vi "Adaptive Channel Equalization.vi"() -> ()   [LabVIEW 2019]
doc: "This example demonstrates how to apply an RLS adaptive filter to channel equalization applications. This example simulates a communication channel with an FIR filter and additional Gaussian noise, simulates the received symbols by applying the FIR filter to the transmitted symbols, and uses an RLS adaptive filter to compensate for the distortion caused by the communication channel. \n\nComplete the following steps to use this example.\n\n1. Select <b>Training</b> from the <b>Mode</b> pull-down menu.\n\n2. Run this example.\n\n3. Observe the <b>Equalizer Output</b> graph until the symbols converge to the four transmitted symbols indicated in the <b>Transmitted Symbols</b> graph.\n\n4. Compare the <b>Equalizer Output</b> and the <b>Received Symbols</b> plot. Notice that the equalizer output converges to the transmitted symbols, whereas the received symbols are difficult to recognize.\n\n5. Select <b>Dicision-Directed</b> from the <b>Mode</b> pull-down menu.\n\n6. Observe the <b>Equalizer Output</b> plot. The equalizer output shows a better convergence."
uses:
  <vilib>/addons/Adaptive Filters/Create/AFT Create FIR RLS (Complex).vi
  <vilib>/addons/Adaptive Filters/Processing/AFT Filter Signal and Update Coefficients (Complex, PtByPt).vi
  <vilib>/addons/Adaptive Filters/Processing/AFT Filter Signal (Complex, PtByPt).vi
  <vilib>/addons/Adaptive Filters/Processing/AFT Update Coefficients (Complex, PtByPt).vi
  <vilib>/addons/Adaptive Filters/NI_AdaptiveFilter.lvlib
panel:
  in  "Tab Control":enum32{"Background", "Scatter Diagram"}(tab)
  in  "Mode":enum16{"Training", "Decision-Directed"}(ring)
  out "Transmitted Symbols":cluster{dbl[], dbl[]}[](graph)
  out "Equalizer Output":cluster{dbl[], dbl[]}[](graph)
  out "Received Symbols":cluster{dbl[], dbl[]}[](graph)
  in  "Filter Length":i32=55 min=2
  in  "Forgetting Factor":dbl=1.0 min=0.0 max=1.0 step=0.0001
  in  "Stop":bool
  # "Refer to the Adaptive Channel Equalization topic in the LabVIEW Help for more information about the background of adaptive channel equalization. Select Help>>Show Context Help and move the cursor over the VI icon of this example for more information."
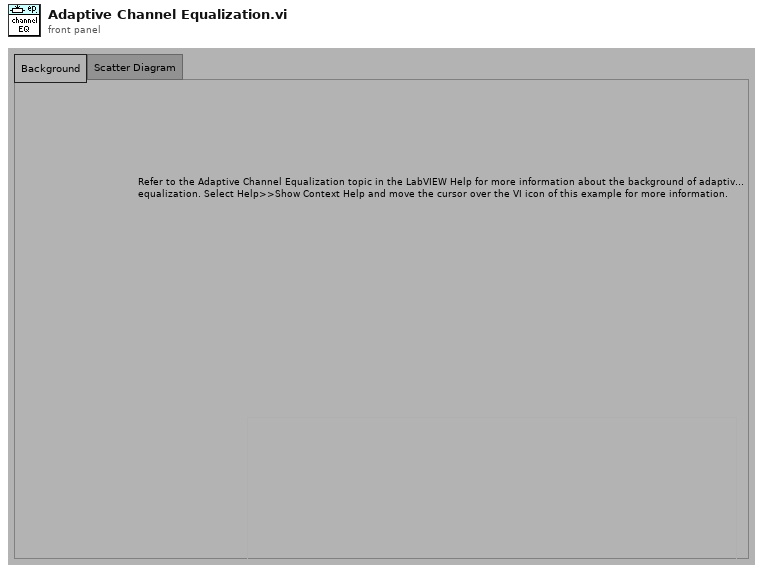
[diagram p1: front panel]
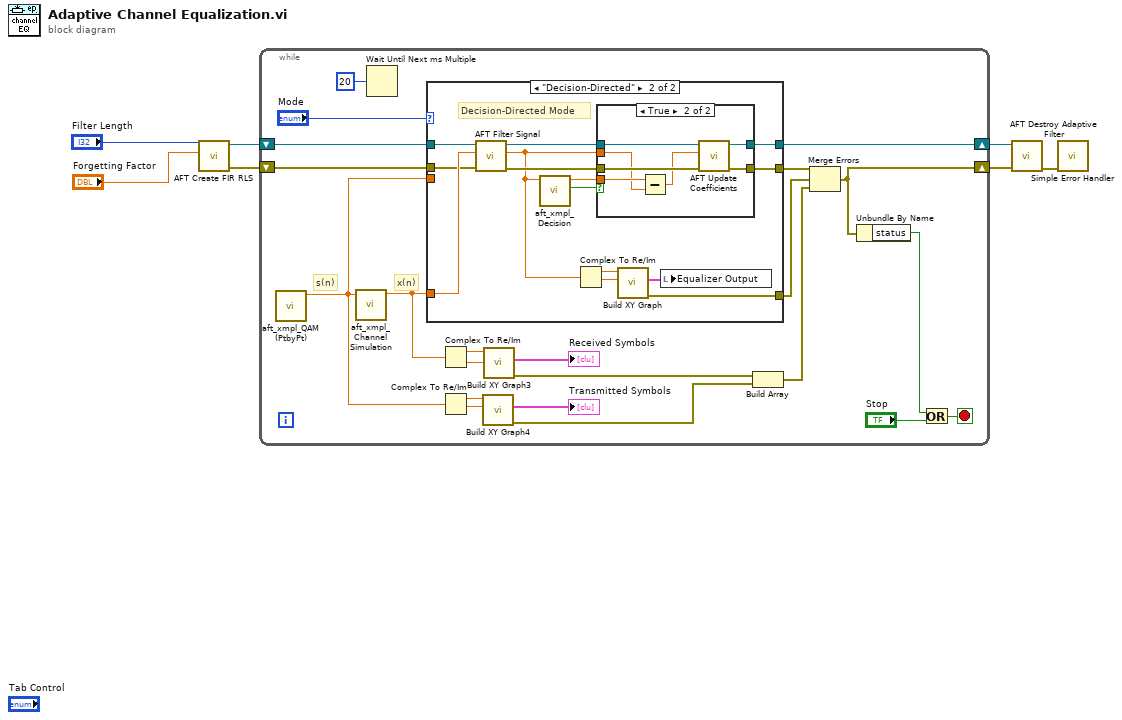
[diagram p0: block diagram]
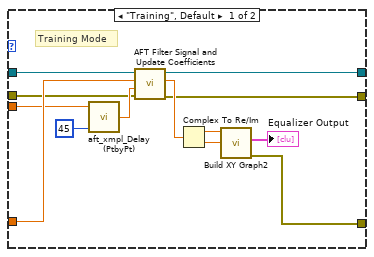
[diagram p2: hidden frame]
diagram:
  n1 = call-poly <vilib>:"AFT Create FIR RLS.vi"("forgetting factor"="Forgetting Factor", "filter length"="Filter Length") -> ("error out"=w3:errorcluster, "adaptive filter out"=w7:refnum<k20>)  [unwired: 2 in, 6 out]
  n2 = while {
    shift-right: [w18] -> w6
    shift-left: w7 -> [w29]
    shift-right: [w11] -> w2
    shift-left: w3 -> [w17]
    stop <- w8 stop-if-true
    # "x(n)"
    # "s(n)"
    n3 = call "aft_xmpl_QAM (PtbyPt).vi"() -> ("QAM signal"=w21:cdb)  [unwired: 11 out]
    n4 = call "aft_xmpl_Channel Simulation.vi"("transmitted signal"=w21) -> ("recieved signal"=w25:cdb)  [unwired: 10 out]
    n5 = Wait Until Next ms Multiple(millisecond multiple=u32 20 ("milliseconds to wait")) -> ()  [unwired: 1 out]
    n6 = case shown="\"Decision-Directed\"" "Mode" {
      tunnel: w29 -> [w42 w52]
      tunnel: [w41 w51] -> w18
      tunnel: w25 -> [w39 w50]
      tunnel: w21 -> [w38 _]
      tunnel: w17 -> [w32 w45]
      tunnel: [w31 w44] -> w16
      tunnel: [w30 w43] -> w12
      frame "Training", Default {
        # "Training Mode"
        n7 = call "aft_xmpl_Delay (PtbyPt).vi"("Delay"=45 ("Delay 2"), "QAM signal"=w38) -> ("shifted x"=w40:cdb)
        n8 = call-poly <vilib>:"AFT Filter Signal and Update Coefficients.vi"("error in (no error)"=w32, "d(n)"=w40, "x(n)"=w39, "adaptive filter in"=w42) -> ("error out"=w31:errorcluster, "y(n)"=w35:cdb, "adaptive filter out"=w41:refnum<k20>)  [unwired: 2 in, 3 out]
        n9 = Complex To Re/Im(x + iy=w35) -> (x=w36:dbl, y=w37:dbl)
        n10 = call "Build XY Graph2"("Y Input"=w37, "X Input"=w36) -> ("error out"=w30:errorcluster, "XY Graph"=→"Equalizer Output":cluster{"Y":dbl[], "Y":dbl[]}[])  [unwired: 3 in, 5 out]
      }
      frame "Decision-Directed" {
        # "Decision-Directed Mode"
        n11 = call-poly <vilib>:"AFT Filter Signal.vi"("error in (no error)"=w45, "x(n)"=w50, "adaptive filter in"=w52) -> ("error out"=w54:errorcluster, "y(n)"=w47:cdb, "adaptive filter out"=w53:refnum<k20>)  [unwired: 1 in, 5 out]
        n12 = call "aft_xmpl_Decision.vi"("y(n)"=w47) -> ("successful?"=w56:bool, "d(n)"=w55:cdb)  [unwired: 9 out]
        n13 = Complex To Re/Im(x + iy=w47) -> (x=w48:dbl, y=w49:dbl)
        n14 = case shown="True" w56 {
          tunnel: w53 -> [w58 w65]
          tunnel: w54 -> [w57 w64]
          tunnel: [w57 w63] -> w44
          tunnel: w55 -> [_ w62]
          tunnel: [w58 w60] -> w51
          tunnel: w47 -> [_ w59]
          frame False {
          }
          frame True {
            n15 = Subtract(x=w62, y=w59) -> (x-y=w61:cdb)
            n16 = call-poly <vilib>:"AFT Update Coefficients.vi"("error in (no error)"=w64, "e(n)"=w61, "adaptive filter in"=w65) -> ("error out"=w63:errorcluster, "adaptive filter out"=w60:refnum<k20>)  [unwired: 1 in, 6 out]
          }
        }
        n17 = call "Build XY Graph"("Y Input"=w49, "X Input"=w48) -> ("error out"=w43:errorcluster, "XY Graph"=w46:cluster{"Y":dbl[], "Y":dbl[]}[])  [unwired: 3 in, 5 out]
        n18 = local write "Equalizer Output"(w46) -> ()
      }
    }
    n19 = Complex To Re/Im(x + iy=w25) -> (x=w27:dbl, y=w26:dbl)
    n20 = Complex To Re/Im(x + iy=w21) -> (x=w22:dbl, y=w23:dbl)
    n21 = call "Build XY Graph4"("Y Input"=w23, "X Input"=w22) -> ("error out"=w14:errorcluster, "XY Graph"=→"Transmitted Symbols":cluster{"Y":dbl[], "Y":dbl[]}[])  [unwired: 3 in, 5 out]
    n22 = call "Build XY Graph3"("Y Input"=w26, "X Input"=w27) -> ("error out"=w15:errorcluster, "XY Graph"=→"Received Symbols":cluster{"Y":dbl[], "Y":dbl[]}[])  [unwired: 3 in, 5 out]
    n23 = Build Array(w15, w14) -> (w13:errorcluster[])
    n24 = Merge Errors(w16, w12, w13) -> (w11:errorcluster)
    n25 = Unbundle By Name(w11) -> ("status"=w10:bool)
    n26 = Or(x=w10, y="Stop") -> (x .or. y?=w8:bool)
  }
  n27 = call <vilib>:"AFT Destroy Adaptive Filter.vi"("error in (no error)"=w2, "adaptive filter in"=w6) -> ("error out"=w1:errorcluster)  [unwired: 9 out]
  n28 = call <vilib>:"Simple Error Handler.vi"("error in (no error)"=w1) -> ()  [unwired: 1 in, 8 out]
